vi "BoolStr2Num.vi"(10 "Boolean string":string) -> (2 "number":i32)   [LabVIEW 2013]
doc: "This VI takes in a string input and outputs a generalized boolean output.\n - \"0\" and \"1\" are mapped to 0,1.\n - Anything else is mapped to 2 (i.e. a variable, blank cell, another number...)."
panel:
  # "Convert boolean string (0, 1, or variable : anything else!)\n to number (0,1,2)."
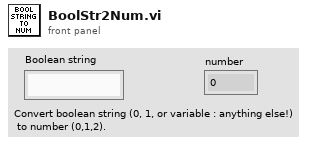
[diagram p1: front panel]
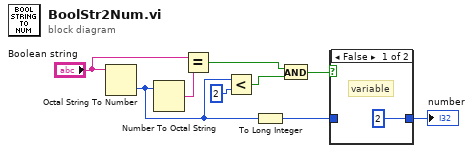
[diagram p0: block diagram]
diagram:
  n1 = Octal String To Number(4:"Boolean string") -> (0:w2:u32)  [unwired: 2 in, 1 out]
  n2 = Number To Octal String(2:w2) -> (0:w9:string)  [unwired: 1 in]
  n3 = Equal?(x="Boolean string", y=w9) -> (x = y?=w4:bool)
  n4 = Less?(x=w2, y=u32 2) -> (x < y?=w5:bool)
  n5 = To Long Integer(number=w2) -> (32bit integer=w1:i32)
  n6 = And(x=w4, y=w5) -> (x .and. y?=w3:bool)
  n7 = case shown="False" w3 {
    tunnel: w1 -> [_ w11]
    tunnel: [2 w11] -> w7
    frame False {
      # "variable"
    }
    frame True {
      # "bool"
    }
  }
  "number" <- w7
